vi "E872_CalibratedMapLightField_MCLS.vi"() -> ()   [LabVIEW 2020]
uses:
  C:/Users/101d/Documents/Princeton Instruments/LightField/Add-in and Automation SDK/Samples/LabVIEW Automation/lightfield-automation-labview/LightField Automation.lvclass
  C:/Program Files (x86)/National Instruments/LabVIEW 2020/instr.lib/DCServoMotor/Thorlabs.MotionControl.Controls.dll
  C:/Program Files (x86)/National Instruments/LabVIEW 2020/instr.lib/DCServoMotor/ThorLabs.MotionControl.KCube.DCServoCLI.dll
panel:
  in  "Number of data points":dbl=3.0
  in  "End Current (mA)":dbl=47.3
  in  "Start Current (mA)":dbl=47.1
  in  "End Position (°):":dbl=80.0 min=0.0 max=360.0
  in  "Step Size (°):":dbl=10.0 min=0.0 max=360.0
  in  "Case Selector":i32
  out "Device":refnum<k24>
  out "reference out":refnum<k24>
  in  "DCServoOn/Off":bool
  out "DCServoRunning":bool
  out "hdl out":i32
  out "LaserRunning":bool
  in  "MCLSOn/Off":bool
  out "error out":errorcluster
  out "Y":dbl
  out "X":dbl
  out "StageRunning":bool
  in  "error in (no error)":errorcluster
  out "LoopCounter":i32
  in  "Return":bool
  in  "stop":bool
  out "Progress":dbl(slide) scale=0.0..1.0
  in  "Start":bool
  in  "Resolution (um):":dbl=5.0
  in  "Map Size (pixels):":i32=6
  out "LFObject":refnum<class "LightField Automation.lvclass">
  in  "Experiment Name:":string="600IRWide"
  out "LFRunning":bool
  in  "LightFieldOn/Off":bool
  out "Calibration":dbl[](array[numeric])
  out "StageChannels":string[](array[string])
  in  "StageOn/Off":bool
  # "STAGE"
  # "LASER"
  # "MOTOR"
  # "LIGHTFIELD"
  # "Motor (rotation):"
  # "Map:"
  # "LightField:"
  # "Power Dependence:"
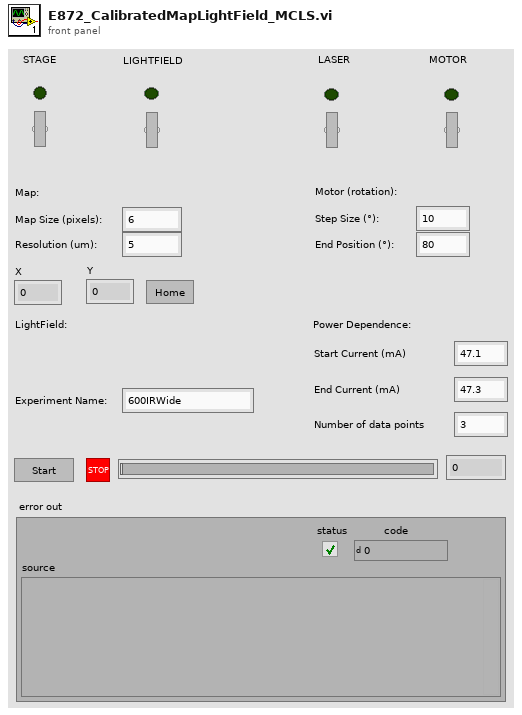
[diagram p1: front panel]
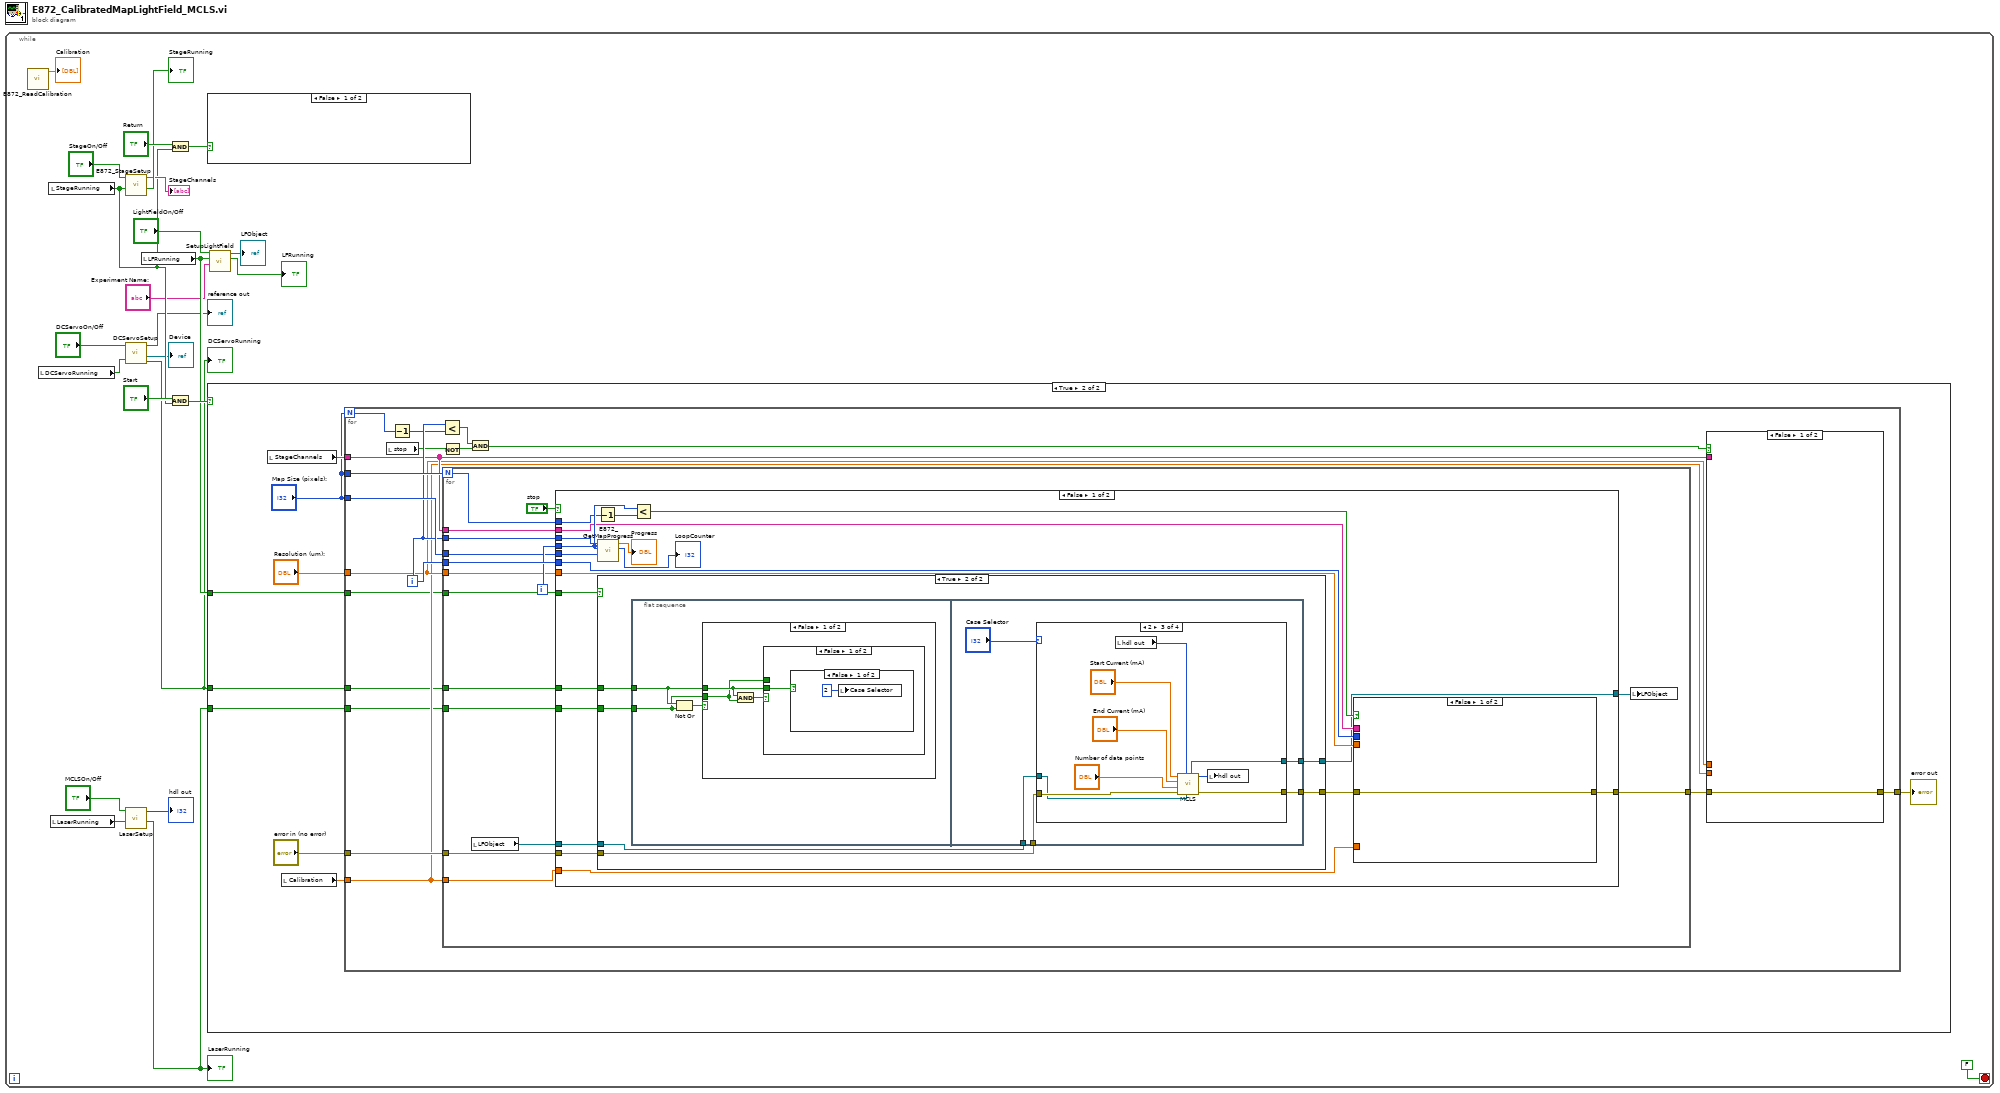
[diagram p0: block diagram]
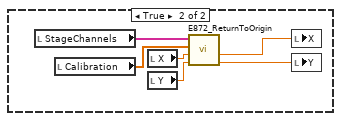
[diagram p2: hidden frame]
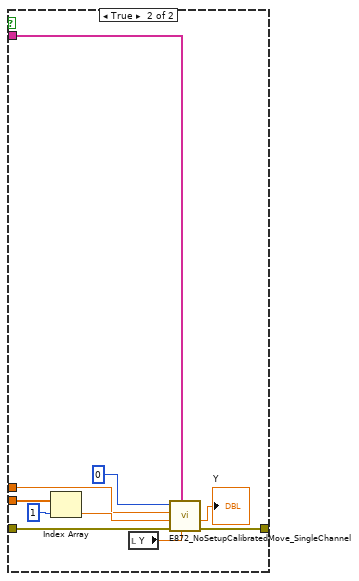
[diagram p4: hidden frame]
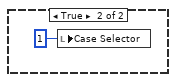
[diagram p6: hidden frame]
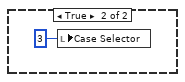
[diagram p7: hidden frame]
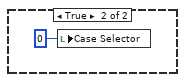
[diagram p8: hidden frame]
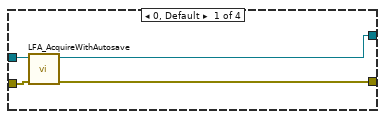
[diagram p9: hidden frame]
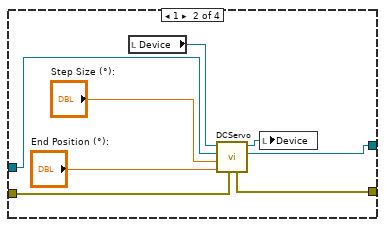
[diagram p10: hidden frame]
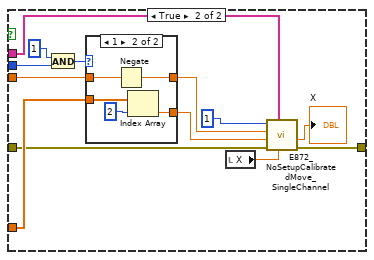
[diagram p12: hidden frame]
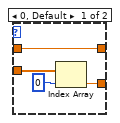
[diagram p13: hidden frame]
diagram:
  n1 = while {
    stop <- FALSE stop-if-true
    n2 = call "E872_ReadCalibration.vi"() -> ("Calibration"=→"Calibration":dbl[])  [unwired: 11 in]
    n3 = local read "DCServoRunning"() -> (w4:bool)
    n4 = local read "StageRunning"() -> (w15:bool)
    n5 = local read "LaserRunning"() -> (w8:bool)
    n6 = call "DCServoSetup.vi"("DCServoOn/Off"="DCServoOn/Off", "DCServoRunningIn"=w4) -> ("reference out"=→"reference out":refnum<k24>, "Device"=→"Device":refnum<k24>, "DCServoRunning"=w2:bool)  [unwired: 3 in]
    "DCServoRunning" <- w2
    n7 = call <instrlib>:"LaserSetup.vi"("LaserRunningIn"=w8, "LaserOn/Off"="MCLSOn/Off") -> ("LaserRunning"=w1:bool, "hdl out"=→"hdl out":i32)  [unwired: 8 in]
    "LaserRunning" <- w1
    n8 = call "E872_StageSetup.vi"("StageRunningIn"=w15, "StageOn/Off"="StageOn/Off") -> ("StageRunningOut"=→"StageRunning":bool, "StageChannels"=→"StageChannels":string[])  [unwired: 8 in]
    n9 = local read "LFRunning"() -> (w13:bool)
    n10 = And(x="Return", y=w15) -> (x .and. y?=w20:bool)
    n11 = And(x="Start", y=w15) -> (x .and. y?=w22:bool)
    n12 = case shown="False" w20 {
      frame False {
      }
      frame True {
        n13 = local read "StageChannels"() -> (w28:string[])
        n14 = local read "Calibration"() -> (w25:dbl[])
        n15 = local read "X"() -> (w27:dbl)
        n16 = local read "Y"() -> (w26:dbl)
        n17 = call "E872_ReturnToOrigin.vi"("Y"=w26, "X"=w27, "Calibration"=w25, "StageChannels"=w28) -> ("Y 2"=w30:dbl, "X 2"=w29:dbl)  [unwired: 6 in]
        n18 = local write "X"(w29) -> ()
        n19 = local write "Y"(w30) -> ()
      }
    }
    n20 = case shown="True" w22 {
      tunnel: w13 -> [_ w36]
      tunnel: w2 -> [_ w32]
      tunnel: w1 -> [_ w31]
      frame False {
      }
      frame True {
        n21 = local read "StageChannels"() -> (w38:string[])
        n22 = local read "Calibration"() -> (w37:dbl[])
        n23 = for {
          N: "Map Size (pixels):" -> [w48]
          tunnel: "Map Size (pixels):" -> [w57]
          tunnel: "Map Size (pixels):" -> [w56]
          tunnel: "error in (no error)" -> [w55]
          tunnel: w38 -> [w53]
          tunnel: w37 -> [w51]
          tunnel: "Resolution (um):" -> [w52]
          tunnel: w36 -> [w50]
          tunnel: [w49] -> w35
          tunnel: w32 -> [w41]
          tunnel: w31 -> [w40]
          i -> [w54]
          n24 = local read "stop"() -> (w42:bool)
          n25 = Decrement(x=w48) -> (x-1=w46:i32)
          n26 = Less?(x=w54, y=w46) -> (x < y?=w44:bool)
          n27 = Not(x=w42) -> (.not. x?=w43:bool)
          n28 = for {
            N: w57 -> [w84]
            tunnel: w54 -> [w83]
            tunnel: w54 -> [w82]
            tunnel: w56 -> [w80]
            tunnel: [w79] -> w47
            tunnel: w55 -> [w74]
            tunnel: w53 -> [w78]
            tunnel: w51 -> [w77]
            tunnel: w52 -> [w76]
            tunnel: w50 -> [w75]
            tunnel: w41 -> [w70]
            tunnel: w40 -> [w69]
            i -> [w81]
            n29 = local read "LFObject"() -> (w72:refnum<class "LightField Automation.lvclass">)
            n30 = case shown="False" "stop" {
              tunnel: w84 -> [w87 _]
              tunnel: w83 -> [w103 _]
              tunnel: w82 -> [w102 _]
              tunnel: w81 -> [w101 _]
              tunnel: w80 -> [w100 _]
              tunnel: [w99 w176] -> w79
              tunnel: w78 -> [w98 _]
              tunnel: w77 -> [w97 _]
              tunnel: w76 -> [w96 _]
              tunnel: w75 -> [w95 _]
              tunnel: w74 -> [w94 w176]
              tunnel: w72 -> [w90 w175]
              tunnel: [w89 w175] -> w71
              tunnel: w70 -> [w86 _]
              tunnel: w69 -> [w85 _]
              frame False {
                n31 = Decrement(x=w87) -> (x-1=w88:i32)
                n32 = call "E872_GetMapProgress.vi"("Map Size (Pixels)"=w100, "j"=w101, "i"=w102) -> ("LoopCounter"=→"LoopCounter":i32, "Progress"=→"Progress":dbl)  [unwired: 7 in]
                n33 = case shown="True" w95 {
                  tunnel: w94 -> [w106 w110]
                  tunnel: [w106 w108] -> w93
                  tunnel: w90 -> [w105 w109]
                  tunnel: [w105 w107] -> w89
                  tunnel: w86 -> [_ w112]
                  tunnel: w85 -> [_ w111]
                  frame False {
                  }
                  frame True {
                    n34 = flat-sequence {
                      tunnel: w112 -> [w114]
                      tunnel: w111 -> [w113]
                      tunnel: w110 -> [w128]
                      tunnel: w109 -> [w127]
                      tunnel: [w126] -> w108
                      tunnel: [w125] -> w107
                      frame #0 {
                        n35 = Not Or(1:w113, 2:w114) -> (0:w115:bool)
                        n36 = case shown="False" w115 {
                          tunnel: w114 -> [w117 _]
                          tunnel: w113 -> [w116 _]
                          frame False {
                            n37 = And(x=w117, y=w116) -> (x .and. y?=w118:bool)
                            n38 = case shown="False" w118 {
                              tunnel: w117 -> [w119 _]
                              tunnel: w116 -> [_ _]
                              frame False {
                                n39 = case shown="False" w119 {
                                frame False {
                                n40 = local write "Case Selector"(2) -> ()
                                }
                                frame True {
                                n41 = local write "Case Selector"(1) -> ()
                                }
                                }
                              }
                              frame True {
                                n42 = local write "Case Selector"(3) -> ()
                              }
                            }
                          }
                          frame True {
                            n43 = local write "Case Selector"(0) -> ()
                          }
                        }
                      }
                      frame #1 {
                        n44 = case shown="2" "Case Selector" {
                          tunnel: w128 -> [w132 w139 w146 w150]
                          tunnel: w127 -> [w131 w140 w144 w151]
                          tunnel: [w130 w138 w145 w150] -> w126
                          tunnel: [w129 w137 w143 w151] -> w125
                          frame 0, Default {
                            n45 = call "LFA_AcquireWithAutosave.vi"("error in (no error)"=w132, "LightField Automation in"=w131) -> ("error out"=w130:errorcluster, "LightField Automation out"=w129:refnum<class "LightField Automation.lvclass">)  [unwired: 7 in, 1 out]
                          }
                          frame 1 {
                            n46 = local read "Device"() -> (w136:refnum<k24>)
                            n47 = call "DCServo.vi"("error in (no error)"=w139, "End Position"="End Position (°):", "Step Size"="Step Size (°):", "LightField Automation in"=w140, "Device"=w136) -> ("LightField Automation out"=w137:refnum<class "LightField Automation.lvclass">, "reference out"=w135:refnum<k24>, "error out"=w138:errorcluster)  [unwired: 4 in]
                            n48 = local write "Device"(w135) -> ()
                          }
                          frame 2 {
                            n49 = local read "hdl out"() -> (w141:i32)
                            n50 = call <instrlib>:"MCLS.vi"("LightField Automation in"=w144, "hdl"=w141, "error in (no error)"=w146, "Number of data points"="Number of data points", "End Current (mA)"="End Current (mA)", "Start Current (mA)"="Start Current (mA)") -> ("error out"=w145:errorcluster, "hdl out"=w142:i32, "LightField Automation out"=w143:refnum<class "LightField Automation.lvclass">)  [unwired: 2 in]
                            n51 = local write "hdl out"(w142) -> ()
                          }
                          frame 3 {
                          }
                        }
                      }
                    }
                  }
                }
                n52 = Less?(x=w101, y=w88) -> (x < y?=w104:bool)
                n53 = case shown="False" w104 {
                  tunnel: w103 -> [_ w163]
                  tunnel: [w152 w153] -> w99
                  tunnel: w93 -> [w152 w154]
                  tunnel: w98 -> [_ w157]
                  tunnel: w97 -> [_ w156]
                  tunnel: w96 -> [_ w155]
                  frame False {
                  }
                  frame True {
                    n54 = And(x=1, y=w163) -> (x .and. y?=w162:i32)
                    n55 = case shown="1" w162 {
                      tunnel: w156 -> [w167 w171]
                      tunnel: [w166 w170] -> w165
                      tunnel: w155 -> [w168 w173]
                      tunnel: [w168 w172] -> w160
                      frame 0, Default {
                        n56 = Index Array(array=w167, index=0) -> (element=w166:dbl)
                      }
                      frame 1 {
                        n57 = Negate(x=w173) -> (-x=w172:dbl)
                        n58 = Index Array(array=w171, index=2) -> (element=w170:dbl)
                      }
                    }
                    n59 = local read "X"() -> (w159:dbl)
                    n60 = call "E872_NoSetupCalibratedMove_SingleChannel.vi"("Starting position"=w159, "PIShift channels 2"=w157, "error in (no error)"=w154, "Calibration (nm/step)"=w165, "Distance (um)"=w160, "Channel"=1) -> ("error out"=w153:errorcluster, "Final Position"=→"X":dbl)  [unwired: 1 in, 1 out]
                  }
                }
              }
              frame True {
              }
            }
            n61 = local write "LFObject"(w71) -> ()
          }
          n62 = And(x=w44, y=w43) -> (x .and. y?=w45:bool)
          n63 = case shown="False" w45 {
            tunnel: w47 -> [w58 w60]
            tunnel: w53 -> [_ w63]
            tunnel: w52 -> [_ w62]
            tunnel: w51 -> [_ w61]
            tunnel: [w58 w59] -> w49
            frame False {
            }
            frame True {
              n64 = Index Array(array=w61, index=1) -> (element=w66:dbl)
              n65 = local read "Y"() -> (w65:dbl)
              n66 = call "E872_NoSetupCalibratedMove_SingleChannel.vi"("Starting position"=w65, "PIShift channels 2"=w63, "error in (no error)"=w60, "Calibration (nm/step)"=w66, "Distance (um)"=w62, "Channel"=0) -> ("error out"=w59:errorcluster, "Final Position"=→"Y":dbl)  [unwired: 1 in, 1 out]
            }
          }
        }
        "error out" <- w35
      }
    }
    n67 = call "SetupLightField.vi"("Experiment Name:"="Experiment Name:", "LFRunningIn"=w13, "LFOn/Off"="LightFieldOn/Off") -> ("LFRunning"=→"LFRunning":bool, "LFObject"=→"LFObject":refnum<class "LightField Automation.lvclass">)  [unwired: 7 in]
  }
